vi "Main.vi"() -> ()   [LabVIEW 2017]
uses:
  Motion Type Def.ctl
panel:
  out "Movement":T1=enum."Triangular"
  out "max V":dbl
  out "Loop Iterations":i32
  out "Displacement Array":dbl[](array[numeric])
  out "Velocity Array":dbl[](array[numeric])
  out "Accel Array":dbl[](array[numeric])
  out "Displacement":dbl[](graph)
  out "Velocity":dbl[](graph)
  out "Acceleration":dbl[](graph)
  out "Motion Planning Outputs":T2
  in  "Motion Planning Inputs":T3
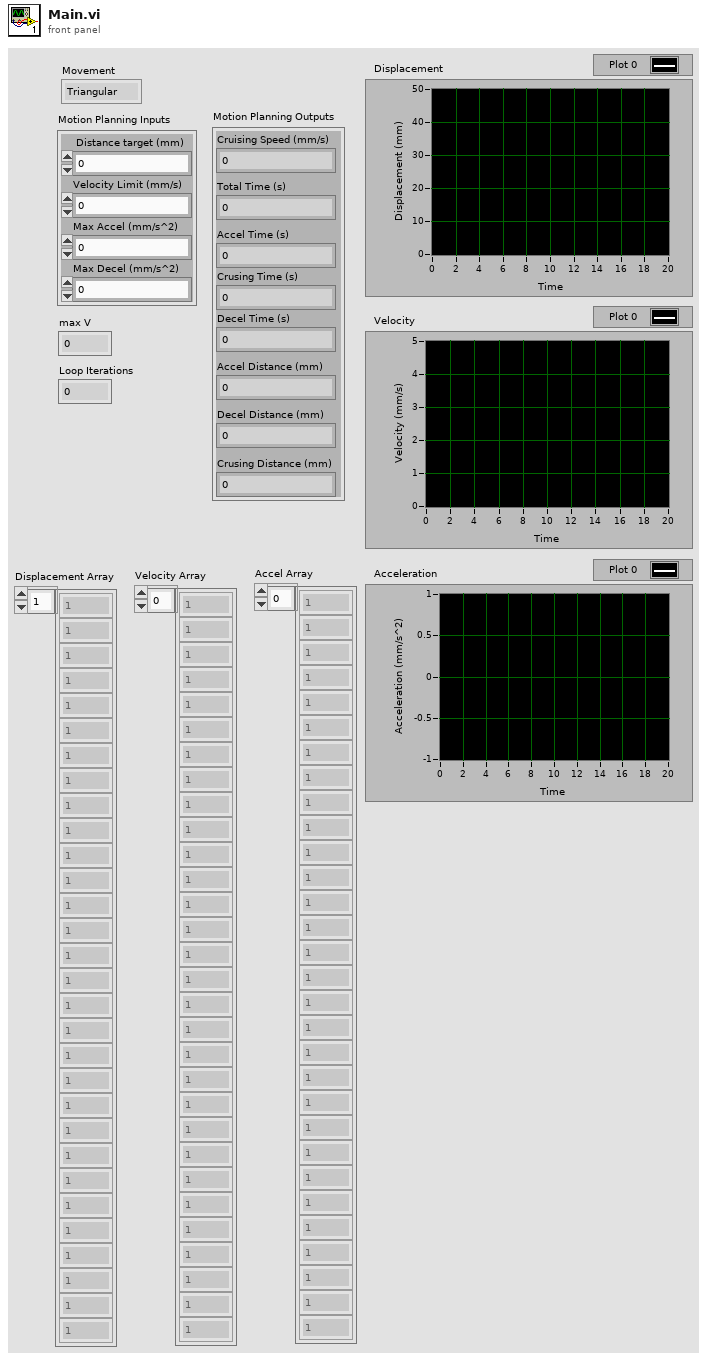
[diagram p1: front panel]
types:
  T1 = typedef "Motion Type Def.ctl" = enum16{"Trapezodial", "Triangular"}
  T2 = cluster{"Cruising Speed (mm/s)":dbl, "Crusing Time (s)":dbl, "Decel Time (s)":dbl, "Accel Time (s)":dbl, "Total Time (s)":dbl, "Accel Distance (mm)":dbl, "Decel Distance (mm)":dbl, "Crusing Distance (mm)":dbl}
  T3 = cluster{" Distance target (mm)":dbl, "Max Accel (mm/s^2)":dbl, "Max Decel (mm/s^2)":dbl, "Velocity Limit (mm/s) ":dbl}
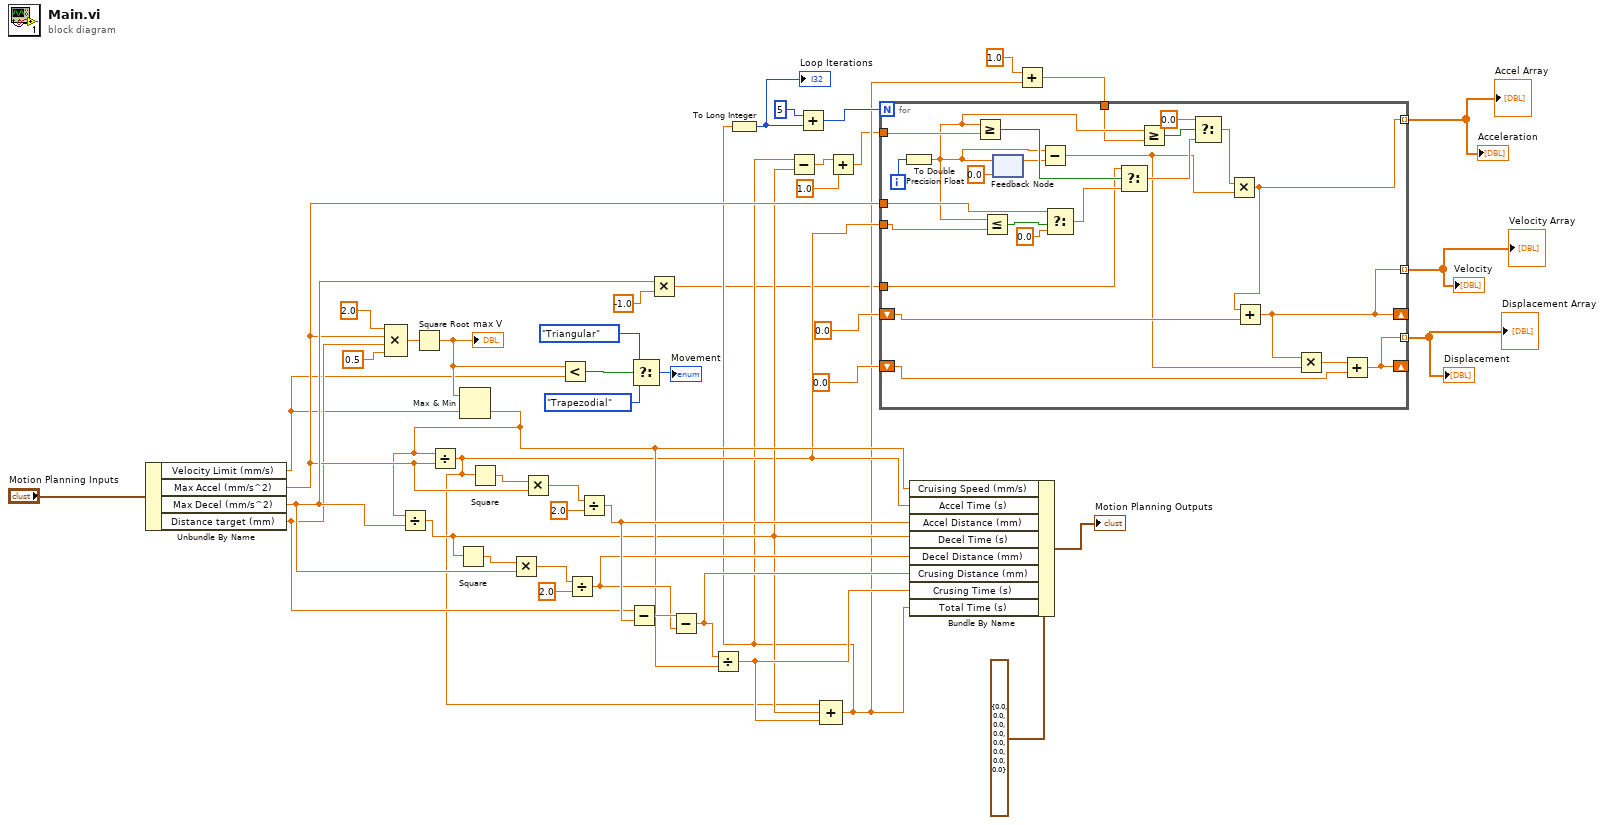
[diagram p0: block diagram]
diagram:
  n1 = Unbundle By Name("Motion Planning Inputs") -> ("Velocity Limit (mm/s)"=w5:dbl, "Max Accel (mm/s^2)"=w21:dbl, "Max Decel (mm/s^2)"=w30:dbl, "Distance target (mm)"=w20:dbl)
  n2 = Compound Arithmetic op=MULTIPLY(2.0 ("value"), w21, w20, 0.5 ("value")) -> (w18:dbl)
  n3 = Square Root(x=w18) -> (sqrt(x)=w6:dbl)
  "max V" <- w6
  n4 = Max & Min(x=w6, y=w5) -> (min(x,y)=w17:dbl)  [unwired: 1 out]
  n5 = Divide(x=w17, y=w30) -> (x/y=w16:dbl)
  n6 = Divide(x=w17, y=w21) -> (x/y=w15:dbl)
  n7 = Square(x=w16) -> (x^2=w33:dbl)
  n8 = Square(x=w15) -> (x^2=w34:dbl)
  n9 = Multiply(x=w33, y=w30) -> (x*y=w32:dbl)
  n10 = Multiply(x=w34, y=w21) -> (x*y=w35:dbl)
  n11 = Less?(x=w6, y=w5) -> (x < y?=w4:bool)
  n12 = Divide(x=w32, y=2.0) -> (x/y=w27:dbl)
  n13 = Divide(x=w35, y=2.0) -> (x/y=w28:dbl)
  n14 = Subtract(x=w20, y=w28) -> (x-y=w29:dbl)
  n15 = Select(t=Motion_Type_Def."Triangular", s=w4, f=Motion_Type_Def."Trapezodial") -> (s? t:f=→"Movement":T1)
  n16 = Multiply(x=w30, y=-1.0) -> (x*y=w11:dbl)
  n17 = Subtract(x=w29, y=w27) -> (x-y=w26:dbl)
  n18 = Divide(x=w26, y=w17) -> (x/y=w25:dbl)
  n19 = Compound Arithmetic op=ADD(w15, w16, w25) -> (w13:dbl)
  n20 = To Long Integer(number=w13) -> (32bit integer=w38:i32)
  "Loop Iterations" <- w38
  n21 = Subtract(x=w13, y=w16) -> (x-y=w14:dbl)
  n22 = Add(x=5, y=w38) -> (x+y=w24:i32)
  n23 = Add(x=w14, y=1.0) -> (x+y=w8:dbl)
  n24 = Bundle By Name(cluster=T2 {"Cruising Speed (mm/s)"=0.0, "Crusing Time (s)"=0.0, "Decel Time (s)"=0.0, "Accel Time (s)"=0.0, "Total Time (s)"=0.0, "Accel Distance (mm)"=0.0, "Decel Distance (mm)"=0.0, "Crusing Distance (mm)"=0.0} ("Motion Planning Outputs 2"), "Cruising Speed (mm/s)"=w17, "Accel Time (s)"=w15, "Accel Distance (mm)"=w28, "Decel Time (s)"=w16, "Decel Distance (mm)"=w27, "Crusing Distance (mm)"=w26, "Crusing Time (s)"=w25, "Total Time (s)"=w13) -> (→"Motion Planning Outputs":T2)
  n25 = Add(x=1.0, y=w13) -> (x+y=w10:dbl)
  n26 = for {
    N: w24 -> [_]
    tunnel: w21 -> [w67]
    tunnel: [w51] -> w41 mode=indexing
    shift-right: [w50] -> _
    shift-left: 0.0 -> [w64]
    tunnel: [w50] -> w40 mode=indexing
    shift-right: [w61] -> _
    shift-left: 0.0 -> [w46]
    tunnel: [w61] -> w39 mode=indexing
    tunnel: w8 -> [w60]
    tunnel: w15 -> [w59]
    tunnel: w10 -> [w56]
    tunnel: w11 -> [w47]
    i -> [w58]
    n27 = To Double Precision Float(number=w58) -> (double precision float=w57:dbl)
    n28 = Greater Or Equal?(x=w57, y=w60) -> (x >= y?=w66:bool)
    n29 = Less Or Equal?(x=w57, y=w59) -> (x <= y?=w69:bool)
    n30 = feedback-in #1(w57) -> ()
    n31 = feedback #1(0.0) -> (w63:dbl)
    n32 = Subtract(x=w57, y=w63) -> (x-y=w49:dbl)
    n33 = Select(t=w67, s=w69, f=0.0) -> (s? t:f=w65:dbl)
    n34 = Select(t=w47, s=w66, f=w65) -> (s? t:f=w53:dbl)
    n35 = Greater Or Equal?(x=w57, y=w56) -> (x >= y?=w55:bool)
    n36 = Select(t=0.0, s=w55, f=w53) -> (s? t:f=w52:dbl)
    n37 = Multiply(x=w52, y=w49) -> (x*y=w51:dbl)
    n38 = Add(x=w51, y=w64) -> (x+y=w50:dbl)
    n39 = Multiply(x=w50, y=w49) -> (x*y=w48:dbl)
    n40 = Add(x=w48, y=w46) -> (x+y=w61:dbl)
  }
  "Acceleration" <- w41
  "Velocity" <- w40
  "Displacement" <- w39
  "Accel Array" <- w41
  "Velocity Array" <- w40
  "Displacement Array" <- w39
